vi "ASIA Pump Handler.vi"   [LabVIEW 2018, in "Support Library.lvlib"]
uses:
  Support Library.lvlib
  <vilib>/addons/_JKI.lib/Serialization/JSON/JKI JSON Serialization.lvlib
  ASIA Pump/Pump Settings.ctl
  ASIA Pump.lvlib
types:
  T1 = typedef "ASIA Pump.lvlib/Pump Settings.ctl" = cluster{"ASIA Pump #":i32, "channel":i32, "Simulated":bool}
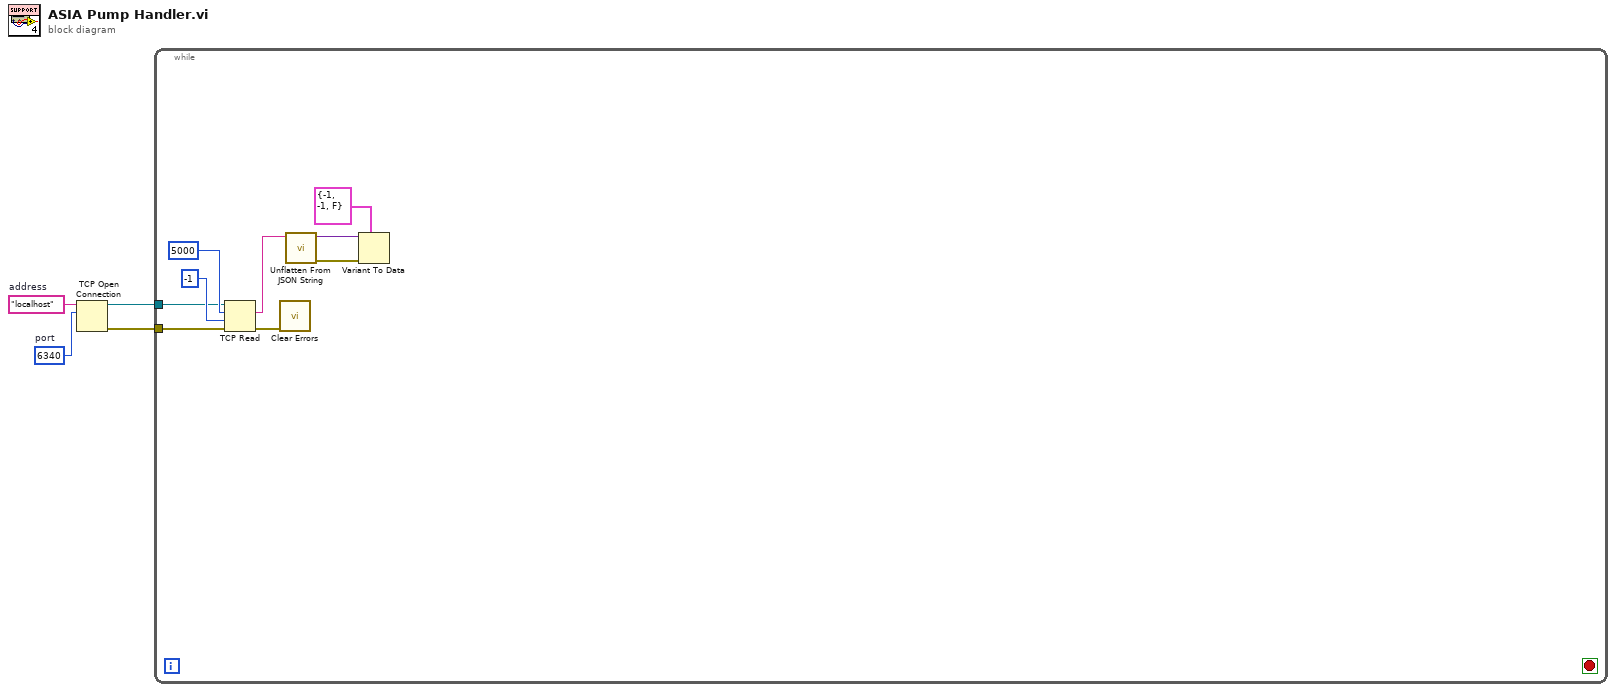
[diagram p0: block diagram]
diagram:
  w4 = u16 6340  # port
  w3 = "localhost"  # address
  n1 = TCP Open Connection(address=w3, remote port or service name=w4) -> (connection ID=w1:refnum<k5>, error out=w2:errorcluster)  [unwired: 3 in]
  n2 = while {
    tunnel: w2 -> [w6]
    tunnel: w1 -> [w5]
    stop <- _ stop-if-true
    n3 = TCP Read(connection ID=w5, bytes to read=5000, error in (no error)=w6, 9:-1 ("timeout ms (25000)")) -> (data out=w8:string, error out=w9:errorcluster)  [unwired: 1 in, 1 out]
    n4 = call <vilib>:"Clear Errors.vi"("error in (no error)"=w9) -> ()  [unwired: 5 in, 2 out]
    n5 = call <vilib>:"Unflatten From JSON String.vi"("JSON String"=w8) -> ("error out"=w12:errorcluster, "Variant"=w13:variant)  [unwired: 9 in]
    n6 = Variant To Data(error in=w12, type=T1 {"ASIA Pump #"=-1, "channel"=-1, "Simulated"=FALSE} ("ASIA Pump C"), Variant=w13) -> ()  [unwired: 2 out]
  }
